vi "test_scd_formatChannelsIntoGetData.vi"(8 "error in (no error)":errorcluster) -> (0 "error out":errorcluster)   [LabVIEW 2020, in "horiba.test.lvlib"]
uses:
  horiba.test.lvlib
  45d4d790-c366-4b76-8c4f-2299ecb11d09.vi
  7cc76bf0-e789-4d30-8454-154dbd193357.vi
  <vilib>/JDP Science/JSONtext/Variant to JSON Text.vi
  <vilib>/JDP Science/JSONtext/Set Item.vi
  <vilib>/addons/_JKI Toolkits/Caraya/classes/Assert/Assert Equal Value_Variant.vi
  <vilib>/addons/_JKI Toolkits/Caraya/classes/Assert/Assert Not Error.vi
  <vilib>/JDP Science/JSONtext/LVClass Serializer/JSONtext LVClass Serializer.lvclass
  <vilib>/addons/_JKI Toolkits/Caraya/classes/Test/Test.lvclass
  <vilib>/JDP Science/JSONtext/JSONtext.lvlib
  <vilib>/addons/_JKI Toolkits/Caraya/classes/Assert/Assert.lvclass
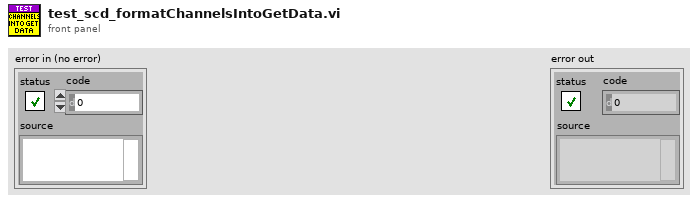
[diagram p1: front panel]
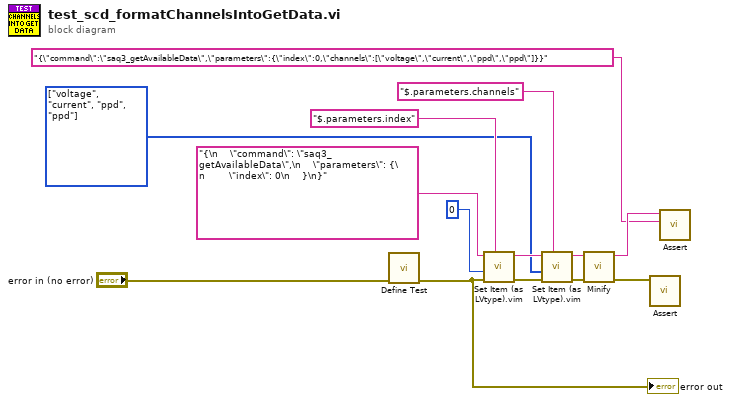
[diagram p0: block diagram]
diagram:
  w9 = enum16{"current", "voltage", "ppd", "photon"}[] [enum."voltage", enum."current", enum."ppd", enum."ppd"] items=["current", "voltage", "ppd", "photon"] ("Array")
  n1 = call <vilib>:"Define Test.vi"("error in (no error)"="error in (no error)") -> ("error out"=w7:errorcluster)  [unwired: 9 in, 1 out]
  "error out" <- w7
  n2 = call "Set Item (as LVtype).vim"("$Path or Item Name"="$.parameters.index", "error in (no error)"=w7, "Anything"=0 ("Index"), "JSON"="{\n    \"command\": \"saq3_getAvailableData\",\n    \"parameters\": {\n        \"index\": 0\n    }\n}") -> ("error out"=w6:errorcluster, "<JSON>"=w10:string)  [unwired: 4 in, 1 out]
  n3 = call "Set Item (as LVtype).vim"("$Path or Item Name"="$.parameters.channels", "error in (no error)"=w6, "Anything"=w9, "JSON"=w10) -> ("error out"=w5:errorcluster, "<JSON>"=w8:string)  [unwired: 4 in, 1 out]
  n4 = call <vilib>:"Minify.vi"("error in (no error)"=w5, "JSON"=w8) -> ("error out"=w2:errorcluster, "<JSON>"=w4:string)  [unwired: 7 in, 1 out]
  n5 = call-poly <vilib>:"Assert.vi"("Not Error?"=w2) -> ()  [unwired: 9 in, 2 out]
  n6 = call-poly <vilib>:"Assert.vi"("Y"="{\"command\":\"saq3_getAvailableData\",\"parameters\":{\"index\":0,\"channels\":[\"voltage\",\"current\",\"ppd\",\"ppd\"]}}" ("<JSON>"), "X"=w4) -> ()  [unwired: 8 in, 2 out]
